vi "Initialize.vi"(0 "Incoming Model Base Interface in":refnum<class "Incoming Model Base Interface.lvclass">, 11 "error in (no error)":errorcluster) -> (4 "Incoming Model Base Interface out":refnum<class "Incoming Model Base Interface.lvclass">, 15 "error out":errorcluster)   [LabVIEW 2023, in "Incoming Model Base Interface.lvlib" / "Incoming Model Base Interface.lvclass"]
uses:
  Incoming Model Base Interface.lvclass
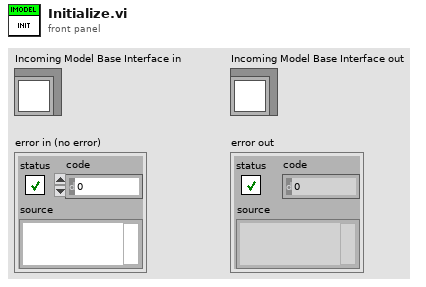
[diagram p1: front panel]
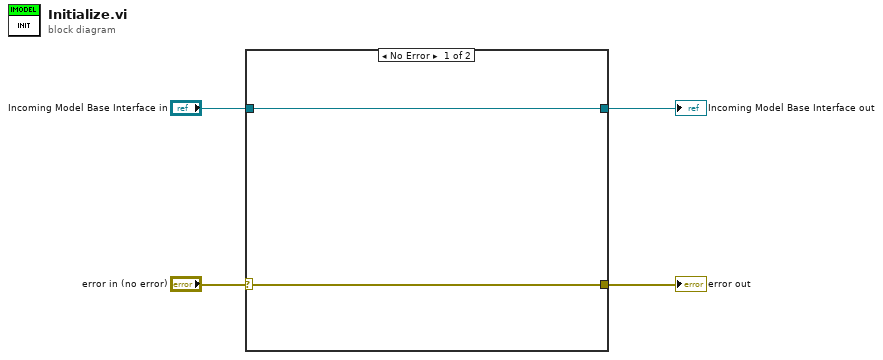
[diagram p0: block diagram]
diagram:
  n1 = case shown="No Error" "error in (no error)" {
    selector: "error in (no error)" -> [w5 w8]
    tunnel: [w5 w8] -> w3
    tunnel: [w6 w7] -> w1
    tunnel: "Incoming Model Base Interface in" -> [w6 w7]
    frame No Error {
    }
    frame Error {
    }
  }
  "error out" <- w3
  "Incoming Model Base Interface out" <- w1
